vi "Scan string for token list.vi"(8 "error in (no error)":errorcluster, 10 "delimiters (space)":string[](array[string])=[" ", "", "", ""], 11 "Query":string) -> (0 "error out":errorcluster, 2 "Tokens":i32, 3 "Token list":string[](array[string]))   [LabVIEW 2013]
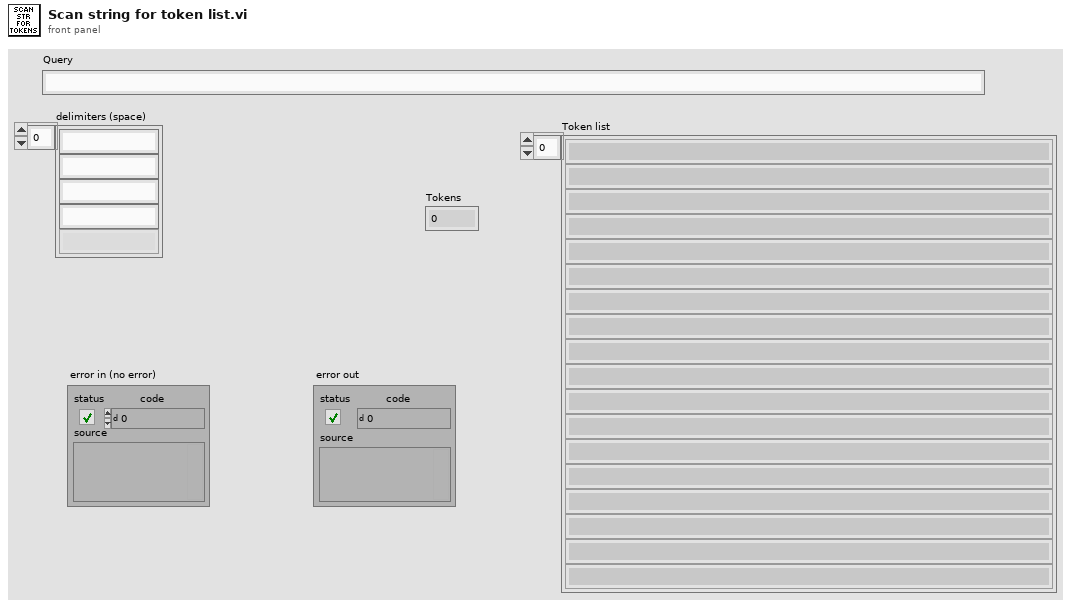
[diagram p1: front panel]
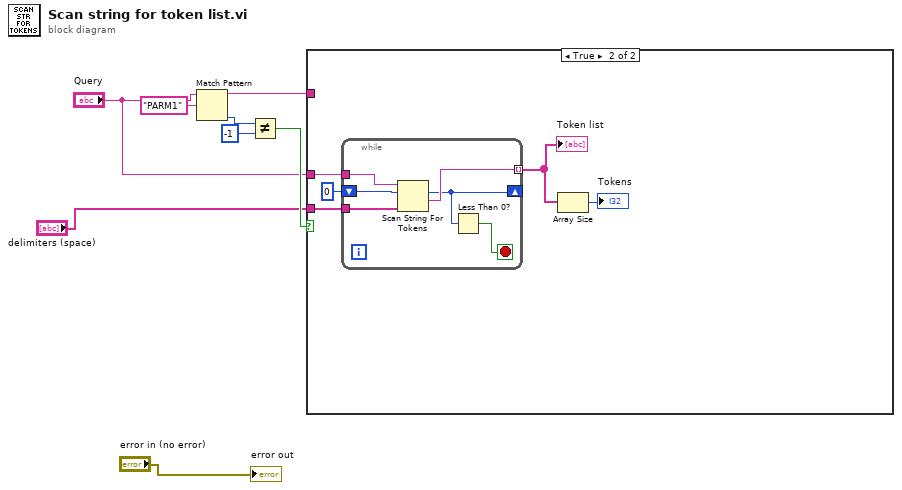
[diagram p0: block diagram]
diagram:
  n1 = Match Pattern(string="Query", regular expression="PARM1") -> (before substring=w4:string, offset past match=w7:i32)  [unwired: 1 in, 2 out]
  n2 = Not Equal?(x=w7, y=-1) -> (x != y?=w5:bool)
  n3 = case shown="True" w5 {
    tunnel: w4 -> [_ _]
    tunnel: "Query" -> [_ w13]
    tunnel: "delimiters (space)" -> [_ w9]
    frame False {
    }
    frame True {
      n4 = while {
        tunnel: w13 -> [w19]
        shift-right: [w15] -> _
        shift-left: 0 ("offset") -> [w18]
        tunnel: [w16] -> w11 mode=indexing
        tunnel: w9 -> [w14]
        stop <- w17 stop-if-true
        n5 = Scan String For Tokens(6:w14, 8:w18, 9:w19) -> (1:w16:string, 2:w15:i32)  [unwired: 3 in, 2 out]
        n6 = Less Than 0?(x=w15) -> (x < 0?=w17:bool)
      }
      "Token list" <- w11
      n7 = Array Size(array=w11) -> (size(s)=→"Tokens":i32)
    }
  }
  "error out" <- "error in (no error)"
